vi "Tosca-2P-Frame Tracking Thread.vi"(2 "IPC":T1, 7 "FrameRate":refnum<vi>) -> (15 "error out":errorcluster)   [LabVIEW 2020]
uses:
  IPC VIs/Tosca-IPC.ctl
  Classes/Parameters/Parameters.lvclass
  Digital Input VIs/Tosca-DI Queue Data.ctl
  Digital Input VIs/Tosca-Input Event.ctl
  Digital Input VIs/Tosca-Input Criterion.ctl
  epl-vi-lib/Utility VIs/Type Defs/Logic State.ctl
  Typedefs/Tosca-Accumulator.ctl
  Typedefs/Tosca-State AODO.ctl
  Typedefs/Tosca-AO Runtime.ctl
  Typedefs/Tosca-DO Runtime.ctl
  epl-vi-lib/Signal Synthesis VIs/4th Generation/Classes/SignalManager/SignalManager.lvclass
  Typedefs/Tosca-Synapse Start Data.ctl
  IPC VIs/Tosca-Message.ctl
  IPC VIs/Tosca-Message Action.ctl
  Typedefs/Tosca-Thread Type.ctl
  Tosca-2P-Notifier Data.ctl
  Typedefs/Tosca-MATLAB Queue Data.ctl
  Visual Stim VIs/Tosca-Grating.ctl
  Visual Stim VIs/Tosca-Grating Type.ctl
  Typedefs/Tosca-File IO Notification.ctl
  Tosca-2P Config.ctl
  Tosca-2P-Globals.vi
  Sub VIs/Tosca-Globals.vi
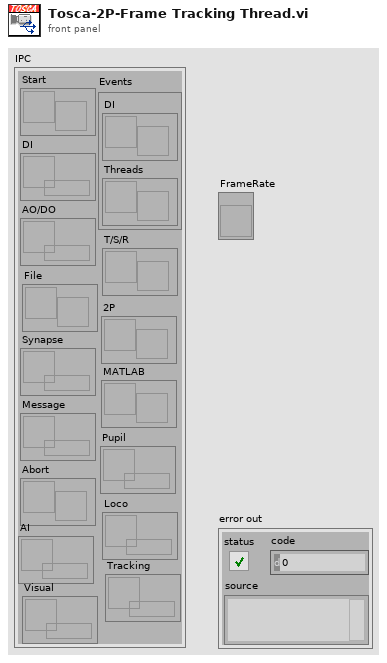
[diagram p1: front panel]
types:
  T1 = typedef "Tosca-IPC.ctl" = cluster{"Start":refnum<notifier>, "DI":refnum<queue>, "AO/DO":refnum<queue>, "Synapse":refnum<queue>, "Message":refnum<queue>, "Abort":refnum<notifier>, "Events":cluster{"DI":refnum<user-event>, "Threads ":refnum<user-event>}, "T/S/R":refnum<notifier>, "2P":refnum<notifier>, "MATLAB":refnum<notifier>, "Pupil":refnum<queue>, "Loco":refnum<queue>, "AI":refnum<queue>, "Tracking":refnum<queue>, "Visual":refnum<queue>, "File":refnum<notifier>}
  T2 = typedef "Tosca-2P Config.ctl" = cluster{"Frame tracker":string, "Terminal":string, "Trigger source":string}
  T3 = typedef "Tosca-Thread Type.ctl" = enum16{"None", "AODO", "Masker", "ET", "Imaging", "Pupil", "AI", "DI", "Camera", "TTL out", "Loco", "Visual"}
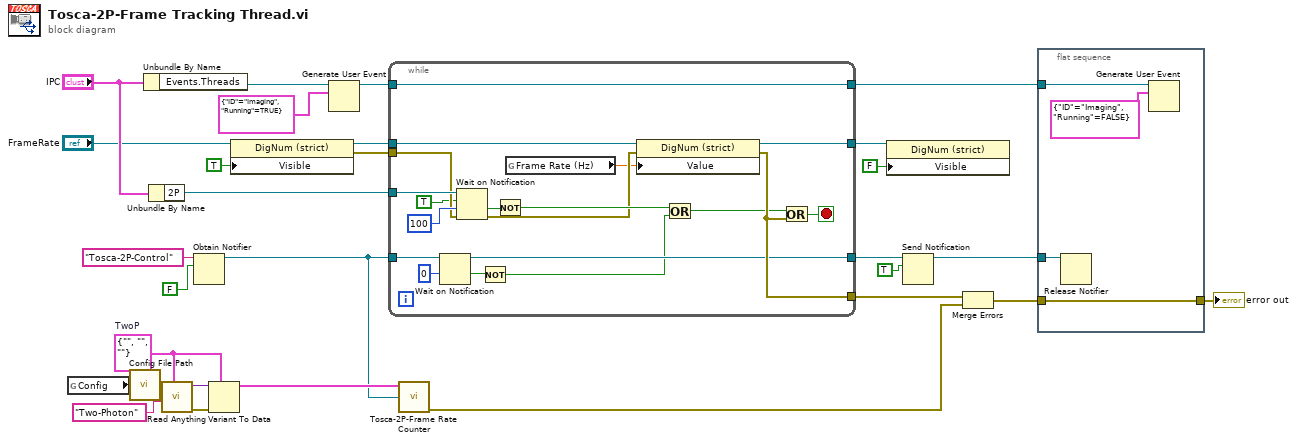
[diagram p0: block diagram]
diagram:
  w15 = T2 {"Frame tracker"="", "Terminal"="", "Trigger source"=""}  # TwoP
  n1 = global read "Tosca-Globals.vi" "Config"() -> (w1:string)
  n2 = call "Config File Path.vi"("AppName"=w1) -> ("Default config file name"=w14:path)
  n3 = Unbundle By Name("IPC") -> ("Events.Threads"=w29:refnum<user-event>)
  n4 = Unbundle By Name("IPC") -> ("2P"=w19:refnum<notifier>)
  n5 = call "Read Anything.vi"("Type of Anything"=w15, "Section Name (Name of \"Type of Anything\")"="Two-Photon" ("Section Name (Name of \"Type of Anything\")"), "Path (dialog)"=w14) -> ("Error Out"=w18:errorcluster, "Anything"=w17:variant)  [unwired: 6 in, 1 out]
  n6 = Obtain Notifier(name (unnamed)="Tosca-2P-Control", notification data type=FALSE) -> (notifier out=w3:refnum<notifier>)  [unwired: 2 in, 2 out]
  n7 = Variant To Data(error in=w18, type=w15, Variant=w17) -> (data=w13:T2)  [unwired: 1 out]
  n8 = property class="DigNum (strict)"(reference="FrameRate", "Visible"=TRUE) -> (reference out=w24:refnum<vi>, error out=w20:errorcluster)  [unwired: 1 in]
  n9 = Generate User Event(user event=w29, event data cluster=cluster{"ID":T3, "Running":bool} {"ID"=enum."Imaging", "Running"=TRUE} ("event data")) -> (user event out=w27:refnum<user-event>)  [unwired: 2 in, 1 out]
  n10 = while {
    tunnel: w27 -> [w48]
    tunnel: [w48] -> w2
    tunnel: w19 -> [w45]
    tunnel: [w37] -> w4
    tunnel: w24 -> [w40]
    tunnel: [w38] -> w22
    tunnel: w20 -> [w42]
    tunnel: w3 -> [w35]
    tunnel: [w34] -> w10
    stop <- w43 stop-if-true
    n11 = Wait on Notification(notifier=w35, timeout in ms (-1)=0) -> (notifier out=w34:refnum<notifier>, timed out?=w32:bool)  [unwired: 2 in, 2 out]
    n12 = Wait on Notification(notifier=w45, ignore previous (F)=TRUE, timeout in ms (-1)=100, error in (no error)=w42) -> (timed out?=w47:bool, error out=w39:errorcluster)  [unwired: 2 out]
    n13 = Not(x=w32) -> (.not. x?=w30:bool)
    n14 = Not(x=w47) -> (.not. x?=w44:bool)
    n15 = global read "Tosca-2P-Globals.vi" "Frame Rate (Hz)"() -> (w36:dbl)
    n16 = property class="DigNum (strict)"(reference=w40, error in=w39, "Value"=w36) -> (reference out=w38:refnum<vi>, error out=w37:errorcluster)
    n17 = Or(x=w44, y=w30) -> (x .or. y?=w31:bool)
    n18 = Or(x=w31, y=w37) -> (x .or. y?=w43:bool)
  }
  n19 = call "Tosca-2P-Frame Rate Counter.vi"("2P"=w13, "2P Control"=w3) -> ("error out"=w8:errorcluster)  [unwired: 13 in]
  n20 = property class="DigNum (strict)"(reference=w22, "Visible"=FALSE) -> ()  [unwired: 1 in, 2 out]
  n21 = Send Notification(notification=TRUE, notifier=w10) -> (notifier out=w6:refnum<notifier>)  [unwired: 1 in, 1 out]
  n22 = Merge Errors(w4, w8) -> (w7:errorcluster)
  n23 = flat-sequence {
    tunnel: w7 -> [w51]
    tunnel: w6 -> [w52]
    tunnel: [w51] -> w5
    tunnel: w2 -> [w49]
    frame #0 {
      n24 = Release Notifier(notifier=w52) -> ()  [unwired: 2 in, 3 out]
      n25 = Generate User Event(user event=w49, event data cluster=cluster{"ID":T3, "Running":bool} {"ID"=enum."Imaging", "Running"=FALSE} ("event data")) -> ()  [unwired: 2 in, 2 out]
    }
  }
  "error out" <- w5
